vi "AddSerDevice.vi"(0 "Handle In":u64[](array[numeric]), 1 "Device ID":u8=1, 2 "Port":string(combo)="COM3", 3 "Baudrate":i32(ring)=19200 items=["4800"=4800, "9600"=9600, "19200"=19200, "38400"=38400, "57600"=57600, "115200"=115200], 4 "Parity":string(combo)="E", 5 "Data Bits":i32(ring)=8 items=["7"=7, "8"=8], 6 "error in (no error)":errorcluster, 7 "Stop Bits":i32(ring)=1 items=["1"=1, "2"=2], 9 "Format":enum32{"RTU", "ASCII"}(ring), 11 "Flow":enum32{"NONE", "RTS/CTS"}(ring)) -> (12 "error out":errorcluster, 14 "Handle Out":u64[](array[numeric]), 15 "Result":i32)   [LabVIEW 2020, in "SnapMB.lvlib"]
uses:
  SnapMB.lvlib
  windows/snapmb.dll
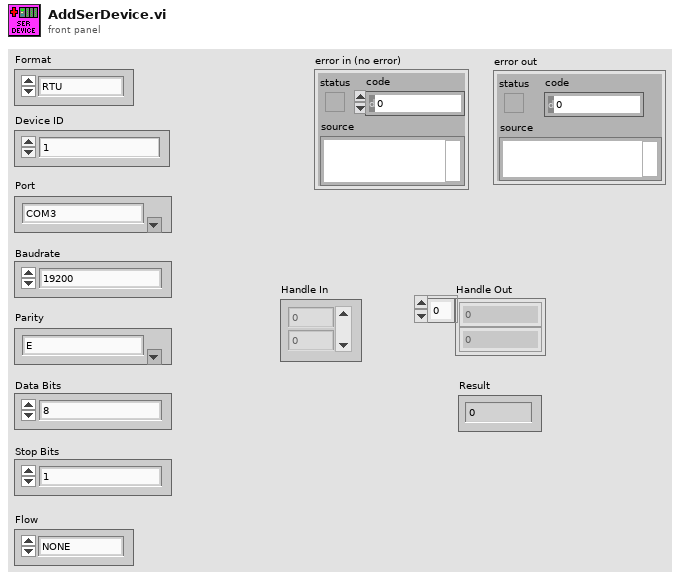
[diagram p1: front panel]
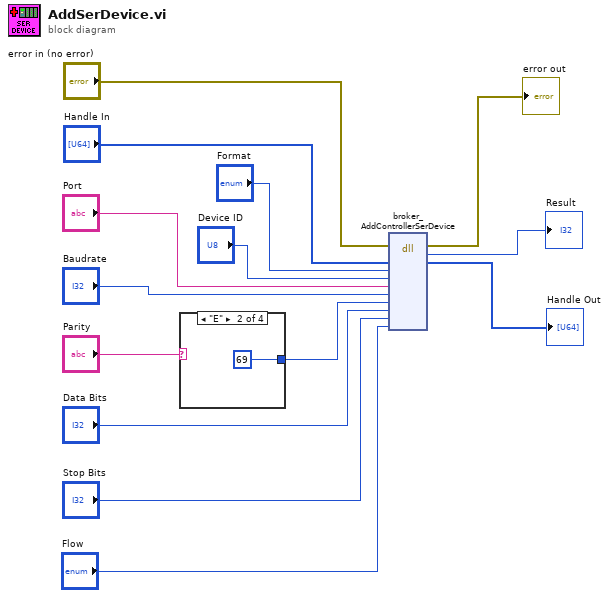
[diagram p0: block diagram]
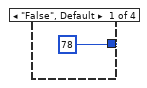
[diagram p2: hidden frame]
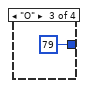
[diagram p3: hidden frame]
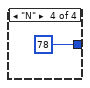
[diagram p4: hidden frame]
diagram:
  n1 = case shown="\"E\"" "Parity" {
    tunnel: [u8 78 u8 69 u8 79 u8 78] -> w6
    frame "False", Default {
    }
    frame "E" {
    }
    frame "O" {
    }
    frame "N" {
    }
  }
  n2 = dll-call lib="D:/SnapMB/LabVIEW/lib/windows/snapmb.dll" fn="broker_AddControllerSerDevice"(error in="error in (no error)", "Handle"="Handle In", "Format"="Format", "DeviceID"="Device ID", "Port"="Port", "Baudrate"="Baudrate", "Parity"=w6, "Data Bits"="Data Bits", "Stop Bits"="Stop Bits", "Flow"="Flow") -> (error out=→"error out":errorcluster, "return type"=→"Result":i32, "Handle"=→"Handle Out":u64[])  [unwired: 10 in, 1 out]
